vi "Set Default (Bool).vi"(8 "error in (no error)":errorcluster, 10 "Default":bool, 11 "Channel in":refnum<class "Channel.lvclass">) -> (0 "error out":errorcluster, 3 "Channel out":refnum<class "Channel.lvclass">)   [LabVIEW 2020, in "VolatusConfig.lvlib" / "Channel.lvclass"]
uses:
  Channel.lvclass
  Channel.lvclass/Channel.ctl
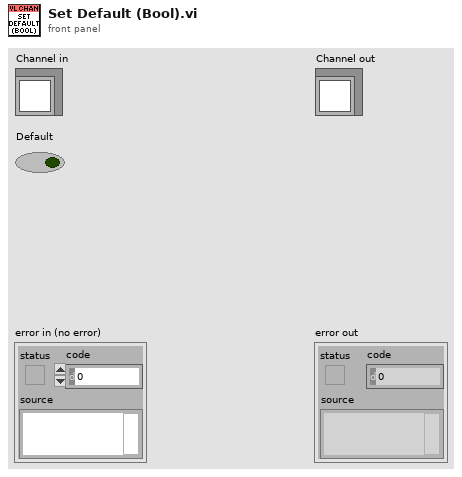
[diagram p1: front panel]
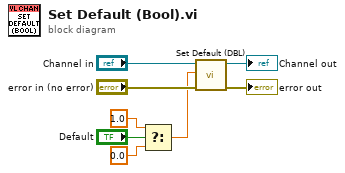
[diagram p0: block diagram]
diagram:
  n1 = Select(t=1.0, s="Default", f=0.0) -> (s? t:f=w2:dbl)
  n2 = call "Set Default (DBL).vi"("error in (no error)"="error in (no error)", "Default"=w2, "Channel in"="Channel in") -> ("error out"=→"error out":errorcluster, "Channel out"=→"Channel out":refnum<class "Channel.lvclass">)  [unwired: 7 in]
